vi "틱카운트.vi"() -> ()   [LabVIEW 2014]
panel:
  out "T 2":dbl
  out "T":dbl
  out "웨이브폼 차트":dbl(graph)
  in  "정지":bool
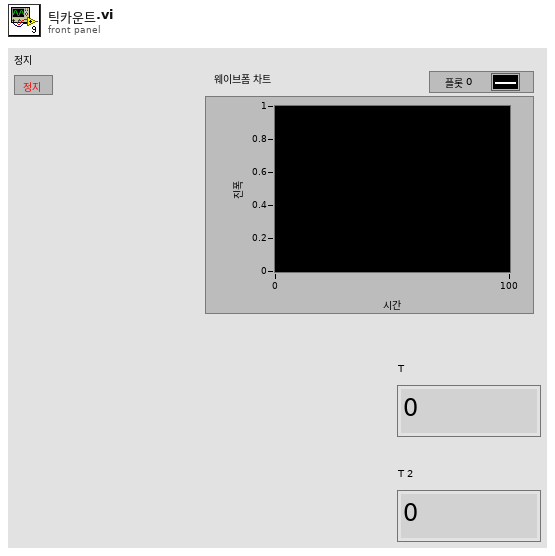
[diagram p1: front panel]
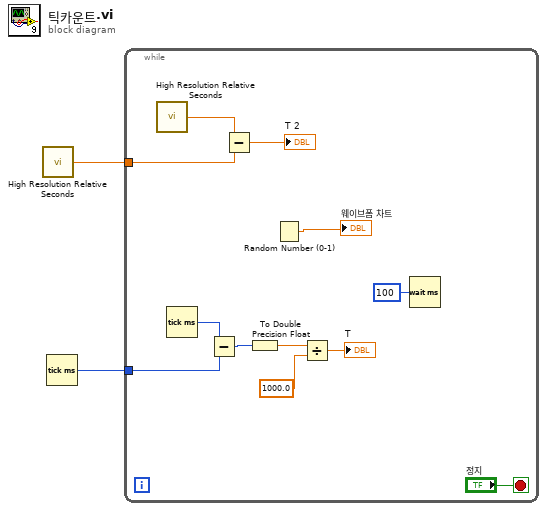
[diagram p0: block diagram]
diagram:
  n1 = call <vilib>:"High Resolution Relative Seconds.vi"() -> ("relative seconds"=w1:dbl)
  n2 = Tick Count (ms)() -> (millisecond timer value=w2:u32)
  n3 = while {
    tunnel: w2 -> [w10]
    tunnel: w1 -> [w4]
    stop <- "정지" stop-if-true
    n4 = call <vilib>:"High Resolution Relative Seconds.vi"() -> ("relative seconds"=w5:dbl)
    n5 = Tick Count (ms)() -> (millisecond timer value=w11:u32)
    n6 = Subtract(x=w11, y=w10) -> (x-y=w9:u32)
    n7 = Subtract(x=w5, y=w4) -> (x-y=→"T 2":dbl)
    n8 = To Double Precision Float(number=w9) -> (double precision float=w8:dbl)
    n9 = Random Number (0-1)() -> (number: 0 to 1=→"웨이브폼 차트":dbl)
    n10 = Divide(x=w8, y=1000.0) -> (x/y=→"T":dbl)
    n11 = Wait (ms)(milliseconds to wait=u32 100 ("대기 시간(ms)")) -> ()  [unwired: 1 out]
  }
